vi "DesiredWheelMovement.vi"(6 "constants":dbl[](array[numeric]), 8 "wheel":T1(ring), 9 "z":dbl, 10 "y":dbl, 11 "x":dbl) -> (2 "desired angle (radians)":dbl, 3 "desired speed":dbl)   [LabVIEW 2013]
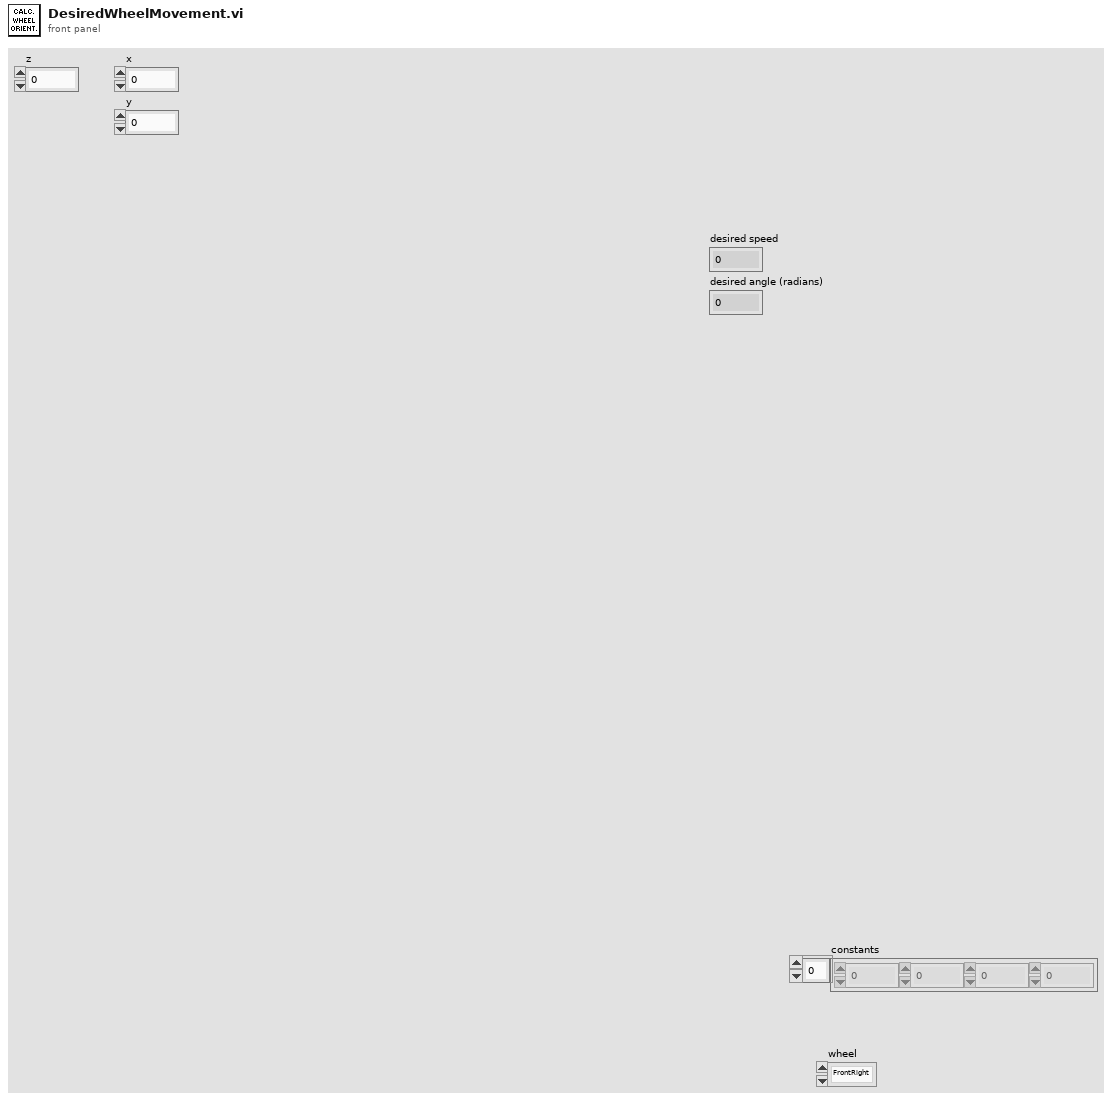
[diagram p1: front panel]
types:
  T1 = enum16{"FrontRight", "FrontLeft", "RearRight", "RearLeft", ""}
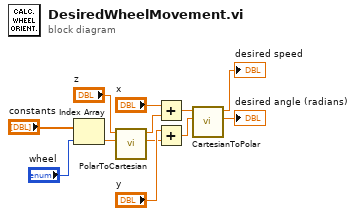
[diagram p0: block diagram]
diagram:
  n1 = Index Array(array="constants", index="wheel") -> (element=w7:dbl)
  n2 = call "PolarToCartesian.vi"("theta (radians)"=w7, "r"="z") -> ("y"=w1:dbl, "x"=w5:dbl)  [unwired: 8 in]
  n3 = Add(x="x", y=w5) -> (x+y=w4:dbl)
  n4 = Add(x="y", y=w1) -> (x+y=w3:dbl)
  n5 = call "CartesianToPolar.vi"("y"=w3, "x"=w4) -> ("theta (radians)"=→"desired angle (radians)":dbl, "r"=→"desired speed":dbl)  [unwired: 8 in]
